vi "HIOKI PW3390 Conf Harmonic.vi"(0 "VISA Resource":refnum<visa-resource-name>, 1 "Set/Query (F: Set)":bool, 5 "Harm Sync (0: U1)":T1(ring), 7 "THD Calc (0: THD-F)":enum16{"F", "R"}(ring), 11 "error in (no error)":errorcluster, 12 "OPC query (T: ON)":bool=TRUE, 13 "Error Out (F: Off)":bool) -> (4 "VISA Resource out":refnum<visa-resource-name>, 6 "Harm Sync out":T1(ring), 8 "THD Calc out":enum16{"F", "R"}(ring), 15 "error out":errorcluster)   [LabVIEW 2009]
doc: "Set/Query\n Set: Send the setting commands for the device.\n Query: Query the setting of the device.\n\nHarm Sync\n Sets the Harmonic Synchronized Source.\n<B>Note</B>\nExt can be set only when the Motor Analysis Option is implemented and when CH B is set to Pulse.\n\nTHD Calc\n Sets the THD Calculation Formula."
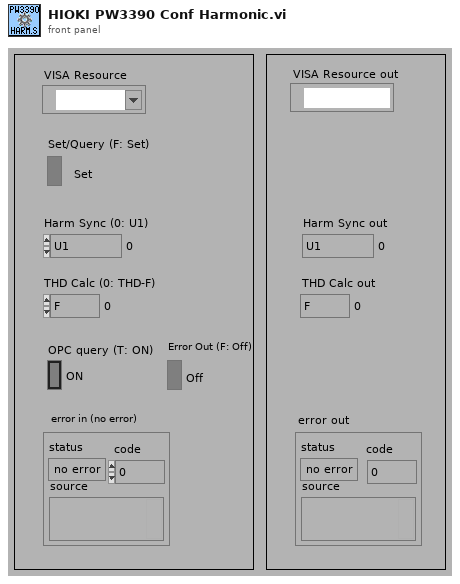
[diagram p1: front panel]
types:
  T1 = enum16{"U1", "U2", "U3", "U4", "I1", "I2", "I3", "I4", "Ext", "DC50ms", "DC100ms"}
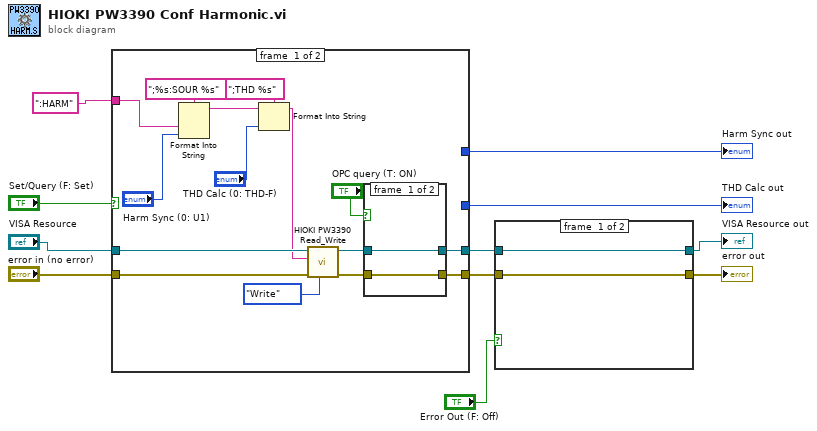
[diagram p0: block diagram]
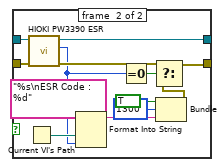
[diagram p2: hidden frame]
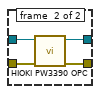
[diagram p3: hidden frame]
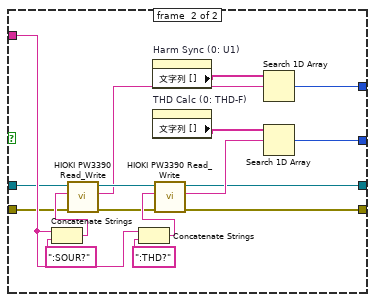
[diagram p4: hidden frame]
diagram:
  n1 = case shown="FALSE" "Set/Query (F: Set)" {
    tunnel: "error in (no error)" -> [w23 w33]
    tunnel: [w12 w39] -> w4
    tunnel: "VISA Resource" -> [w24 w34]
    tunnel: [w13 w40] -> w5
    tunnel: ":HARM" -> [w18 w35]
    tunnel: [_ w48] -> w8
    tunnel: [_ w37] -> w7
    frame #0 {
      n2 = Format Into String(format string=";%s:SOUR %s", w18, "Harm Sync (0: U1)") -> (resulting string=w21:string)  [unwired: 2 in, 1 out]
      n3 = Format Into String(format string=";THD %s", initial string=w21, "THD Calc (0: THD-F)") -> (resulting string=w20:string)  [unwired: 1 in, 1 out]
      n4 = call <instrlib>:"HIOKI PW3390 Read_Write.vi"("Read/Write"=enum16{"Read", "Write"}."Write", "error in (no error)"=w23, "data in"=w20, "VISA Resource"=w24) -> ("error out"=w14:errorcluster, "VISA Resource out"=w15:refnum<visa-resource-name>)  [unwired: 5 in, 1 out]
      n5 = case shown="TRUE" "OPC query (T: ON)" {
        tunnel: [w28 w32] -> w13
        tunnel: [w27 w31] -> w12
        tunnel: w15 -> [w28 w30]
        tunnel: w14 -> [w27 w29]
        frame #0 {
        }
        frame #1 {
          n6 = call <instrlib>:"HIOKI PW3390 OPC.vi"("error in (no error)"=w29, "VISA Resource"=w30) -> ("error out"=w31:errorcluster, "VISA Resource out"=w32:refnum<visa-resource-name>)  [unwired: 7 in, 1 out]
        }
      }
    }
    frame #1 {
      n7 = Concatenate Strings(w35, ":SOUR?") -> (w43:string)
      n8 = call <instrlib>:"HIOKI PW3390 Read_Write.vi"("error in (no error)"=w33, "data in"=w43, "VISA Resource"=w34) -> ("error out"=w41:errorcluster, "data out"=w36:string, "VISA Resource out"=w42:refnum<visa-resource-name>)  [unwired: 6 in]
      n9 = Concatenate Strings(w35, ":THD?") -> (w47:string)
      n10 = property on="Harm Sync (0: U1)" class="Enum (strict)"() -> ("文字列 []"=w38:string[])  [unwired: 2 in, 2 out]
      n11 = property on="THD Calc (0: THD-F)" class="Enum (strict)"() -> ("文字列 []"=w46:string[])  [unwired: 2 in, 2 out]
      n12 = call <instrlib>:"HIOKI PW3390 Read_Write.vi"("error in (no error)"=w41, "data in"=w47, "VISA Resource"=w42) -> ("error out"=w39:errorcluster, "data out"=w45:string, "VISA Resource out"=w40:refnum<visa-resource-name>)  [unwired: 6 in]
      n13 = Search 1D Array(1D array=w38, element=w36) -> (index of element=w37:i32)  [unwired: 1 in]
      n14 = Search 1D Array(1D array=w46, element=w45) -> (index of element=w48:i32)  [unwired: 1 in]
    }
  }
  "THD Calc out" <- w8
  "Harm Sync out" <- w7
  n15 = case shown="TRUE" "Error Out (F: Off)" {
    tunnel: w5 -> [w51 w64]
    tunnel: w4 -> [w50 w63]
    tunnel: [w50 w53] -> w3
    tunnel: [w51 w62] -> w2
    frame #0 {
    }
    frame #1 {
      n16 = Current VI's Path() -> (path=w60:path)
      n17 = call <instrlib>:"HIOKI PW3390 ESR.vi"("error in (no error)"=w63, "VISA Resource"=w64) -> ("error out"=w54:errorcluster, "Output Value"=w52:u8, "VISA Resource out"=w62:refnum<visa-resource-name>)  [unwired: 6 in, 1 out]
      n18 = Format Into String(format string="%s\nESR Code : %d", w60, w52) -> (resulting string=w56:string)  [unwired: 2 in, 1 out]
      n19 = Equal To 0?(x=w52) -> (x = 0?=w61:bool)
      n20 = Bundle("status"=TRUE, "code"=1300, w56) -> (w55:cluster{"status":bool, "code":i32, string})  [unwired: 1 in]
      n21 = Select(t=w54, s=w61, f=w55) -> (s? t:f=w53:errorcluster)
    }
  }
  "error out" <- w3
  "VISA Resource out" <- w2
